vi "SingleBoard_LEDs to Display.vi"(0 "Model Select":T1, 7 "Justice League SingleBoard Map":T9) -> (8 "JL Display":T2={"SSD"="", "Cycle Selection"=enum."Cycle 0", "Bar Selection"=enum."Bar 1", "Temp Setting"=enum."High", "Dryness Level"=enum."Extra Dry", "Time Setting"=enum."Default Time 5", "Dryer Status"=enum."Status 6", "Start/Pause"=FALSE, "Pause"=FALSE, "Control Lock"=FALSE, "Sensing"=FALSE, "Clean Filter"=FALSE, "My Cycle"=FALSE, "Delay Dry"=FALSE, "Volume"=FALSE, "Damp Alert"=FALSE, "Ext Tumble"=FALSE, "Decrement"=FALSE, "Increment"=FALSE, "eDry"=FALSE, "Extra Status"=FALSE})   [LabVIEW 2016]
uses:
  type defs/SB_LEDs.ctl
  type defs/JL Display.ctl
  type defs/Cycle Selection Enum.ctl
  type defs/Bar Enum.ctl
  type defs/Temp Setting Enum.ctl
  type defs/Dryness Enum.ctl
  type defs/Time Enum.ctl
  type defs/Status Enum.ctl
  type defs/JL_Trans-Model.ctl
  <vilib>/Utility/error.llb/whitespace.ctl
  type defs/JL_Trans-state.ctl
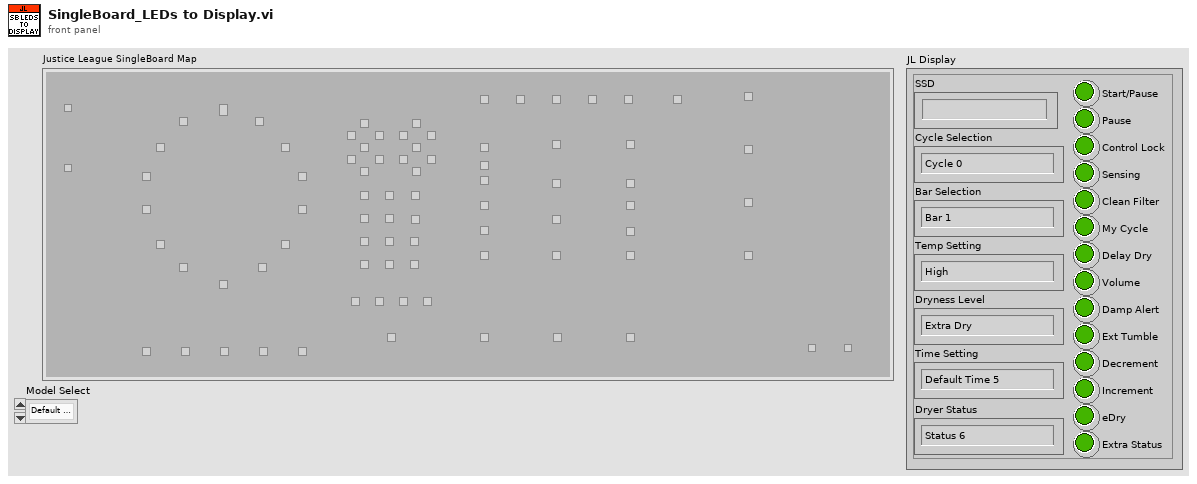
[diagram p1: front panel]
types:
  T1 = typedef "JL_Trans-Model.ctl" = enum16{"Default Model"}
  T2 = typedef "JL Display.ctl" = cluster{"SSD":string, "Cycle Selection":T3, "Bar Selection":T4, "Temp Setting":T5, "Dryness Level":T6, "Time Setting":T7, "Dryer Status":T8, "Start/Pause":bool, "Pause":bool, "Control Lock":bool, "Sensing":bool, "Clean Filter":bool, "My Cycle":bool, "Delay Dry":bool, "Volume":bool, "Damp Alert":bool, "Ext Tumble":bool, "Decrement":bool, "Increment":bool, "eDry":bool, "Extra Status":bool}
  T3 = typedef "Cycle Selection Enum.ctl" = enum16{"Cycle 0", "Cycle 1", "Cycle 2", "Cycle 3", "Cycle 4", "Cycle 5", "Cycle 6", "Cycle 7", "Cycle 8", "Cycle 9", "Cycle 10", "Cycle 11", "Cycle 12", "Cycle 13", "Off", "*Invalid"}
  T4 = typedef "Bar Enum.ctl" = enum16{"Bar 1", "Bar 2", "Bar 3", "Bar 4", "Bar 5", "Off", "*Incorrect*"}
  T5 = typedef "Temp Setting Enum.ctl" = enum16{"Off", "No Heat", "Extra Low", "Low", "Medium", "High", "*Incorrect*"}
  T6 = typedef "Dryness Enum.ctl" = enum16{"Off", "Damp", "Less Dry", "Dry", "More Dry", "Extra Dry", "*Incorrect*"}
  T7 = typedef "Time Enum.ctl" = enum16{"Off", "Default Time 1", "Default Time 2", "Default Time 3", "Default Time 4", "Default Time 5", "*Incorrect*"}
  T8 = typedef "Status Enum.ctl" = enum16{"Status 1", "Status 2", "Status 3", "Status 4", "Status 5", "Status 6", "Off", "*Incorrect*"}
  T9 = typedef "SB_LEDs.ctl" = cluster{"Z101 - Start/Pause":bool, "Z - unpop?":bool, "Z103 - Encoder 0":bool, "Z104 - Encoder 13":bool, "Z105 - Encoder 12":bool, "Z106 - Encoder 11":bool, "Z107 - Encoder 10":bool, "Z108 - Encoder 09":bool, "Z109 - Encoder 08":bool, "Z110 - Encoder 07":bool, "Z111 - Encoder 06":bool, "Z112 - Encoder 05":bool, "Z113 - Encoder 04":bool, "Z114 - Encoder 03":bool, "Z115 - Encoder 02":bool, "Z116 - Encoder 01":bool, "Z117 - Bar 1":bool, "Z118 - Bar 2":bool, "Z119 - Bar 3":bool, "Z120 - Bar 4":bool, "Z121 - Bar 5":bool, "Z122 - SSD1:A":bool, "Z123 - SSD1:B":bool, "Z124 - SSD1:C":bool, "Z125 - SSD1:D":bool, "Z126 - SSD1:E":bool, "Z127 - SSD1:F":bool, "Z128 - SSD1:G":bool, "Z129 - SSD2:A":bool, "Z130 - SSD2:B":bool, "Z131 - SSD2:C":bool, "Z132 - SSD2:D":bool, "Z133 - SSD2:E":bool, "Z134 - SSD2:F":bool, "Z135 - SSD2:G":bool, "Z136 - Pause 2":bool, "Z137 - Pause 3":bool, "Z138 - Control Lock 1":bool, "Z139 - Control Lock 2":bool, "Z140 - Control Lock 3":bool, "Z142 - Sensing 1":bool, "Z142 -Sensing 2":bool, "Z143 - Sensing 3":bool, "Z144 - Extra Status 1":bool, "Z145 - Extra Status 2":bool, "Z146 - Extra Status 3":bool, "Z147 - Extra Status 4":bool, "Z148 - Status 1":bool, "Z149 - Status 2":bool, "Z150 - Status 3":bool, "Z151 - Status 4":bool, "Z152 - Status 5":bool, "Z153 - Status 6":bool, "Z154 - Default Time 5":bool, "Z155 - Default Time 4":bool, "Z153 - Default Time 3":bool, "Z157 -Default Time 2":bool, "Z158 - Default Time 1":bool, "Z159 - Default Time 0":bool, "Z160 - More Dry":bool, "Z161 - Dry":bool, "Z162 - Less Dry":bool, "Z163 - Damp":bool, "Z164 - High":bool, "Z165 - Medium":bool, "Z166 - Extra Low":bool, "Z167 - No Heat":bool, "Z168 - Volume":bool, "Z169 - Damp Alert":bool, "Z170 - Extended Tumble":bool, "Z171 - Time Decrement":bool, "Z172 - Time Increment":bool, "Z173 - eDry":bool, "Z174 -My Cycle":bool, "Z175 - Delay Dry":bool, "Z176 - Clean Lint Filter 1":bool, "Z177 - Clean Lint Filter 2":bool, "Z178 - Clean Lint Filter 3":bool, "Z179 - Pause 1":bool, "OFF - OFF":bool, "MAX - MAX":bool, "Z165B -Low":bool}
  T10 = typedef "JL_Trans-state.ctl" = enum16{"Temp ", "Time", "Level", "stop"}
  T11 = typedef "whitespace.ctl" = u16
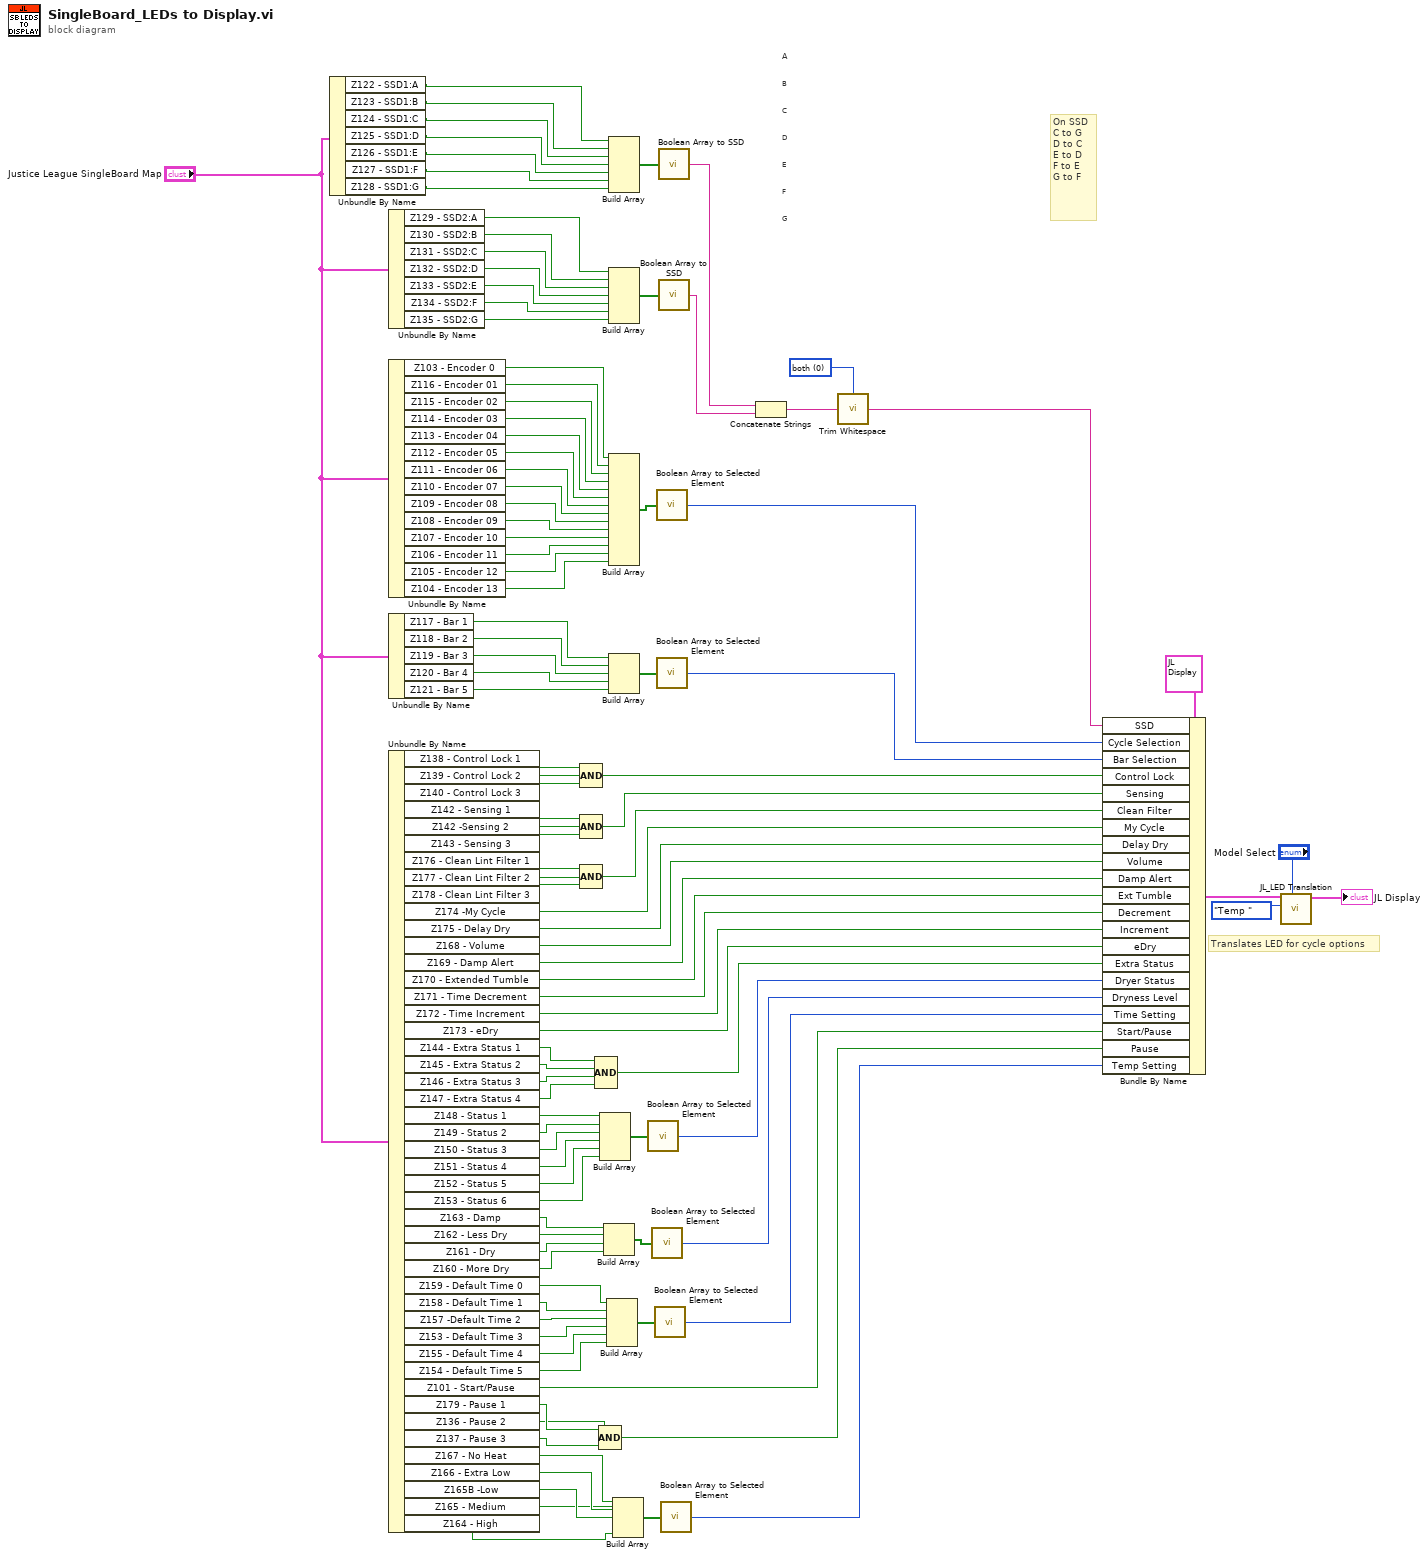
[diagram p0: block diagram]
diagram:
  w13 = T11 0 items=["both", "start of string", "end of string"] ("location (both)")
  # "G"
  # "F"
  # "E"
  # "D"
  # "C"
  # "B"
  # "A"
  # "On SSD \nC to G \nD to C \nE to D\nF to E\nG to F"
  # "Translates LED for cycle options"
  n1 = Unbundle By Name("Justice League SingleBoard Map") -> ("Z122 - SSD1:A"=w7:bool, "Z123 - SSD1:B"=w6:bool, "Z124 - SSD1:C"=w5:bool, "Z125 - SSD1:D"=w4:bool, "Z126 - SSD1:E"=w3:bool, "Z127 - SSD1:F"=w2:bool, "Z128 - SSD1:G"=w1:bool)
  n2 = Unbundle By Name("Justice League SingleBoard Map") -> ("Z129 - SSD2:A"=w109:bool, "Z130 - SSD2:B"=w108:bool, "Z131 - SSD2:C"=w107:bool, "Z132 - SSD2:D"=w106:bool, "Z133 - SSD2:E"=w105:bool, "Z134 - SSD2:F"=w104:bool, "Z135 - SSD2:G"=w103:bool)
  n3 = Unbundle By Name("Justice League SingleBoard Map") -> ("Z103 - Encoder 0"=w100:bool, "Z116 - Encoder 01"=w99:bool, "Z115 - Encoder 02"=w98:bool, "Z114 - Encoder 03"=w97:bool, "Z113 - Encoder 04"=w96:bool, "Z112 - Encoder 05"=w95:bool, "Z111 - Encoder 06"=w94:bool, "Z110 - Encoder 07"=w93:bool, "Z109 - Encoder 08"=w92:bool, "Z108 - Encoder 09"=w91:bool, "Z107 - Encoder 10"=w90:bool, "Z106 - Encoder 11"=w89:bool, "Z105 - Encoder 12"=w88:bool, "Z104 - Encoder 13"=w66:bool)
  n4 = Unbundle By Name("Justice League SingleBoard Map") -> ("Z117 - Bar 1"=w87:bool, "Z118 - Bar 2"=w86:bool, "Z119 - Bar 3"=w85:bool, "Z120 - Bar 4"=w84:bool, "Z121 - Bar 5"=w83:bool)
  n5 = Unbundle By Name("Justice League SingleBoard Map") -> ("Z138 - Control Lock 1"=w80:bool, "Z139 - Control Lock 2"=w79:bool, "Z140 - Control Lock 3"=w78:bool, "Z142 - Sensing 1"=w77:bool, "Z142 -Sensing 2"=w76:bool, "Z143 - Sensing 3"=w75:bool, "Z176 - Clean Lint Filter 1"=w74:bool, "Z177 - Clean Lint Filter 2"=w73:bool, "Z178 - Clean Lint Filter 3"=w72:bool, "Z174 -My Cycle"=w61:bool, "Z175 - Delay Dry"=w60:bool, "Z168 - Volume"=w59:bool, "Z169 - Damp Alert"=w58:bool, "Z170 - Extended Tumble"=w57:bool, "Z171 - Time Decrement"=w56:bool, "Z172 - Time Increment"=w55:bool, "Z173 - eDry"=w54:bool, "Z144 - Extra Status 1"=w52:bool, "Z145 - Extra Status 2"=w51:bool, "Z146 - Extra Status 3"=w50:bool, "Z147 - Extra Status 4"=w53:bool, "Z148 - Status 1"=w47:bool, "Z149 - Status 2"=w46:bool, "Z150 - Status 3"=w45:bool, "Z151 - Status 4"=w44:bool, "Z152 - Status 5"=w43:bool, "Z153 - Status 6"=w42:bool, "Z163 - Damp"=w39:bool, "Z162 - Less Dry"=w38:bool, "Z161 - Dry"=w37:bool, "Z160 - More Dry"=w36:bool, "Z159 - Default Time 0"=w33:bool, "Z158 - Default Time 1"=w32:bool, "Z157 -Default Time 2"=w31:bool, "Z153 - Default Time 3"=w30:bool, "Z155 - Default Time 4"=w29:bool, "Z154 - Default Time 5"=w28:bool, "Z101 - Start/Pause"=w26:bool, "Z179 - Pause 1"=w25:bool, "Z136 - Pause 2"=w24:bool, "Z137 - Pause 3"=w23:bool, "Z167 - No Heat"=w19:bool, "Z166 - Extra Low"=w18:bool, "Z165B -Low"=w17:bool, "Z165 - Medium"=w16:bool, "Z164 - High"=w15:bool)
  n6 = Compound Arithmetic op=AND(w80, w79, w78) -> (w65:bool)
  n7 = Compound Arithmetic op=AND(w77, w76, w75) -> (w63:bool)
  n8 = Compound Arithmetic op=AND(w74, w73, w72) -> (w62:bool)
  n9 = Compound Arithmetic op=AND(w52, w51, w50, w53) -> (w49:bool)
  n10 = Compound Arithmetic op=AND(w25, w24, w23) -> (w22:bool)
  n11 = Build Array(w47, w46, w45, w44, w43, w42) -> (w48:bool[])
  n12 = Build Array(w39, w38, w37, w36) -> (w40:bool[])
  n13 = Build Array(w33, w32, w31, w30, w29, w28) -> (w34:bool[])
  n14 = Build Array(w7, w6, w5, w4, w3, w2, w1) -> (w68:bool[])
  n15 = Build Array(w109, w108, w107, w106, w105, w104, w103) -> (w102:bool[])
  n16 = Build Array(w100, w99, w98, w97, w96, w95, w94, w93, w92, w91, w90, w89, w88, w66) -> (w81:bool[])
  n17 = Build Array(w87, w86, w85, w84, w83) -> (w82:bool[])
  n18 = Build Array(w19, w18, w17, w16, w15) -> (w21:bool[])
  n19 = call "Boolean Array to Selected Element.vi"("Bool Array In"=w48) -> ("Selected Element Out"=w41:i32)  [unwired: 14 in]
  n20 = call "Boolean Array to Selected Element.vi"("Bool Array In"=w40) -> ("Selected Element Out"=w35:i32)  [unwired: 14 in]
  n21 = call "Boolean Array to Selected Element.vi"("Bool Array In"=w34) -> ("Selected Element Out"=w27:i32)  [unwired: 14 in]
  n22 = call "Boolean Array to Selected Element.vi"("Bool Array In"=w81) -> ("Selected Element Out"=w70:i32)  [unwired: 14 in]
  n23 = call "Boolean Array to Selected Element.vi"("Bool Array In"=w82) -> ("Selected Element Out"=w71:i32)  [unwired: 14 in]
  n24 = call "Boolean Array to SSD.vi"("7 Segment Bool Array In"=w68) -> ("7 Segment Out"=w67:string)  [unwired: 14 in]
  n25 = call "Boolean Array to SSD.vi"("7 Segment Bool Array In"=w102) -> ("7 Segment Out"=w101:string)  [unwired: 14 in]
  n26 = call "Boolean Array to Selected Element.vi"("Bool Array In"=w21) -> ("Selected Element Out"=w20:i32)  [unwired: 14 in]
  n27 = Concatenate Strings(w67, w101) -> (w69:string)
  n28 = call <vilib>:"Trim Whitespace.vi"("string"=w69, "location (both)"=w13) -> ("trimmed string"=w14:string)
  n29 = Bundle By Name(cluster=T2 {"SSD"="", "Cycle Selection"=enum."Cycle 0", "Bar Selection"=enum."Bar 1", "Temp Setting"=enum."High", "Dryness Level"=enum."Extra Dry", "Time Setting"=enum."Default Time 5", "Dryer Status"=enum."Status 6", "Start/Pause"=FALSE, "Pause"=FALSE, "Control Lock"=FALSE, "Sensing"=FALSE, "Clean Filter"=FALSE, "My Cycle"=FALSE, "Delay Dry"=FALSE, "Volume"=FALSE, "Damp Alert"=FALSE, "Ext Tumble"=FALSE, "Decrement"=FALSE, "Increment"=FALSE, "eDry"=FALSE, "Extra Status"=FALSE} ("JL Display"), "SSD"=w14, "Cycle Selection"=w70, "Bar Selection"=w71, "Control Lock"=w65, "Sensing"=w63, "Clean Filter"=w62, "My Cycle"=w61, "Delay Dry"=w60, "Volume"=w59, "Damp Alert"=w58, "Ext Tumble"=w57, "Decrement"=w56, "Increment"=w55, "eDry"=w54, "Extra Status"=w49, "Dryer Status"=w41, "Dryness Level"=w35, "Time Setting"=w27, "Start/Pause"=w26, "Pause"=w22, "Temp Setting"=w20) -> (w12:T2)
  n30 = call "JL_LED Translation.vi"("Model Select"="Model Select", "Option"=JL_Trans-state."Temp ", "JL Display"=w12) -> ("JL Display 2"=→"JL Display":T2)  [unwired: 7 in, 1 out]
